vi "Update User Details.vi"(8 "error in (no error)":errorcluster, 10 "Update Credential":T1, 11 "Access in":refnum<class "Access.lvclass">) -> (0 "error out":errorcluster, 3 "Access out":refnum<class "Access.lvclass">)   [LabVIEW 2016, in "Database.lvlib" / "Access.lvclass"]
uses:
  Access.lvclass
  DB/Update Credential.ctl
  DB/Credential.ctl
  Database.lvlib
  User Interface/User Interface.lvlib
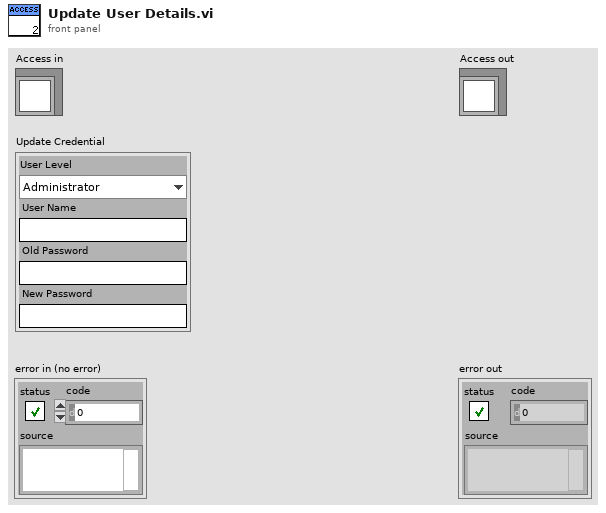
[diagram p1: front panel]
types:
  T1 = typedef "Database.lvlib/Update Credential.ctl" = cluster{"User Level":enum16{"Administrator", "Engineer", "Operator"}, "User Name":string, "Old Password":string, "New Password":string}
  T2 = typedef "Database.lvlib/Credential.ctl" = cluster{"User Level":enum16{"Administrator", "Engineer", "Operator"}, "User Name":string, "Password":string}
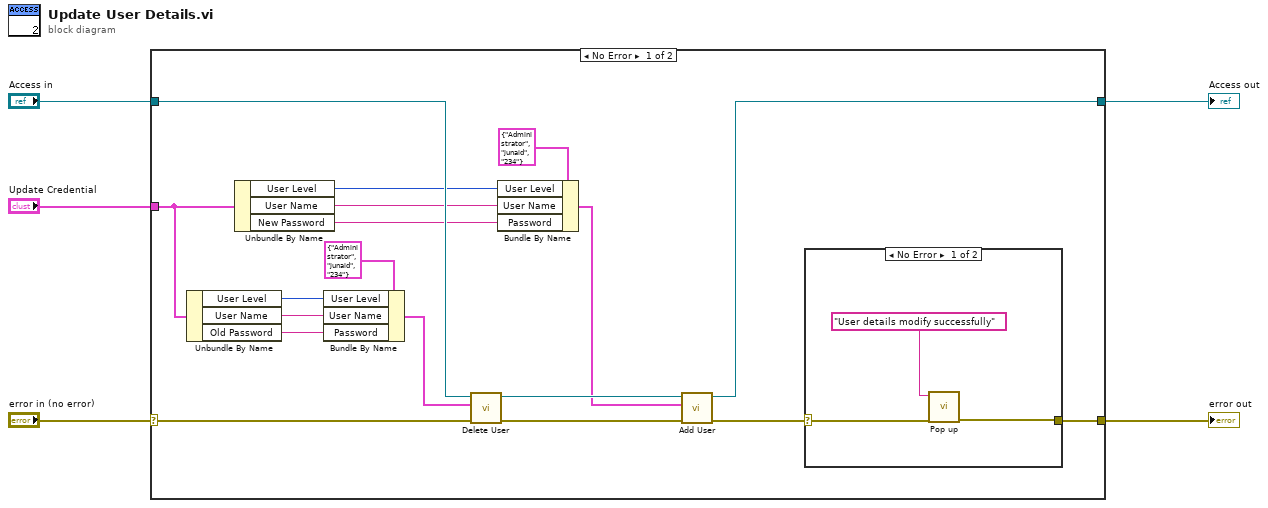
[diagram p0: block diagram]
diagram:
  n1 = case shown="No Error" "error in (no error)" {
    selector: "error in (no error)" -> [w23 w28]
    tunnel: "Access in" -> [w22 w29]
    tunnel: [w19 w29] -> w3
    tunnel: [w6 w28] -> w2
    tunnel: "Update Credential" -> [w13 _]
    frame No Error {
      n2 = Unbundle By Name(w13) -> ("User Level"=w18:enum16{"Administrator", "Engineer", "Operator"}, "User Name"=w17:string, "Old Password"=w16:string)
      n3 = Unbundle By Name(w13) -> ("User Level"=w12:enum16{"Administrator", "Engineer", "Operator"}, "User Name"=w11:string, "New Password"=w10:string)
      n4 = Bundle By Name(cluster=T2 {"User Level"=enum."Administrator", "User Name"="junaid", "Password"="234"} ("Credential"), "User Level"=w18, "User Name"=w17, "Password"=w16) -> (w15:T2)
      n5 = call-dynamic "Delete User.vi"("error in (no error)"=w23, "Credential"=w15, "Access in"=w22) -> ("error out"=w20:errorcluster, "Access out"=w21:refnum<class "Access.lvclass">)  [unwired: 7 in]
      n6 = Bundle By Name(cluster=T2 {"User Level"=enum."Administrator", "User Name"="junaid", "Password"="234"} ("Credential"), "User Level"=w12, "User Name"=w11, "Password"=w10) -> (w9:T2)
      n7 = call-dynamic "Add User.vi"("error in (no error)"=w20, "Credential"=w9, "Access in"=w21) -> ("error out"=w7:errorcluster, "Access out"=w19:refnum<class "Access.lvclass">)  [unwired: 7 in]
      n8 = case shown="No Error" w7 {
        selector: w7 -> [w26 w27]
        tunnel: [w25 w27] -> w6
        frame No Error {
          n9 = call "Pop up.vi"("error in (no error)"=w26, "Message In"="User details modify successfully") -> ("error out"=w25:errorcluster)  [unwired: 9 in]
        }
        frame Error {
        }
      }
    }
    frame Error {
    }
  }
  "error out" <- w2
  "Access out" <- w3
